vi "extract ROI.vi"(7 "ROI Descriptor":T2 {"Contours"."Type" items=["No Selection", "Point", "Line", "Rectangle", "Oval", "Polygon", "Freehand Region", "Annulus", "Unused2", "Unused3", "Broken Line", "Freehand Line", "Rotated Rectangle"]}, 10 "ROI ref in":T1, 11 "CCD image ref":T1) -> (0 "ROI SIZE":i32, 1 "Centroid XY":cluster{"X Centroid":sgl, "Y Centroid":sgl} {"Y Centroid" format="%.2f"; "X Centroid" format="%.2f"}, 3 "img_out":dbl[][](array[numeric]), 4 "Y_base":sgl, 6 "X_base":sgl)   [LabVIEW 2017]
doc: "本VI的作用是将已有的ROI提取出图像，计算出图心，然后在图心上标记ROI的序号。\n本VI对ROI的实际尺寸不敏感，可以随意修改。\n本VI由于最终要出图给camera window，因此不建议并行多分支执行，最好是先执行完，后续提取出来的图再分成各个分支并行执行。"
uses:
  <vilib>/vision/Image Controls.llb/IMAQ Image.ctl
  <vilib>/vision/NI_Vision_Development_Module.lvlib
  <vilib>/ptbypt/NI_PtbyPt.lvlib
  <vilib>/Analysis/NI_AALBase.lvlib
  <vilib>/Analysis/Matrix/NI_Matrix.lvlib
  <vilib>/Analysis/Matrix/Numeric/Multiply/Multiply - RM,R.vi
  <vilib>/Analysis/baseanly.llb/Normalize Matrix.vi
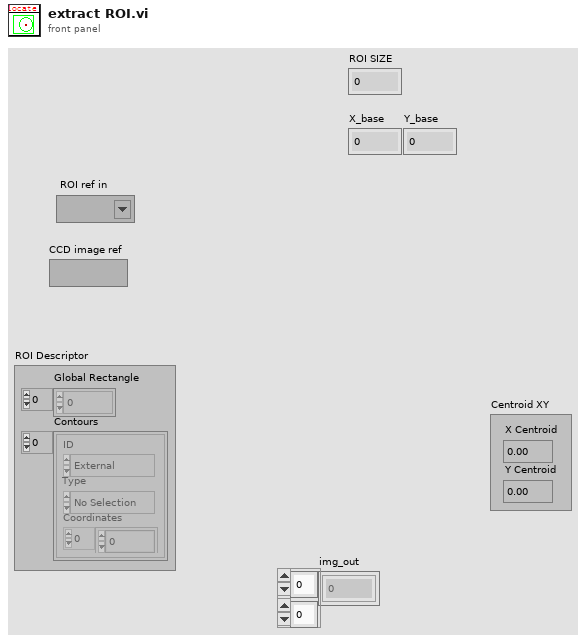
[diagram p1: front panel]
types:
  T1 = typedef "IMAQ Image.ctl" = refnum<image>
  T2 = typedef "ROI Descriptor" = cluster{"Global Rectangle":i32[], "Contours":cluster{"ID":enum32{"External", "Internal"}, "Type":u32, "Coordinates":i32[]}[]}
  T3 = typedef "IMAQ Rectangle" = cluster{"Left":i32, "Top":i32, "Right":i32, "Bottom":i32, "Rotation":dbl}
  T4 = typedef "NI_Matrix.lvlib/RealMatrix.ctl" = dbl[][]
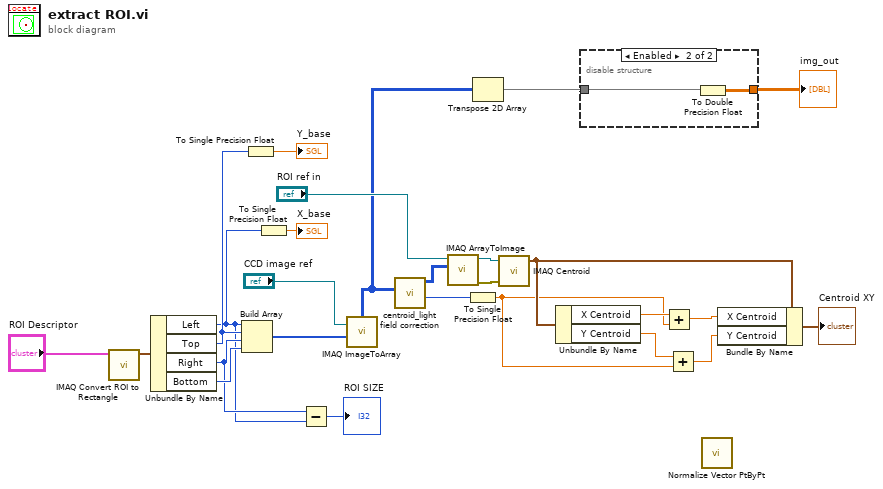
[diagram p0: block diagram]
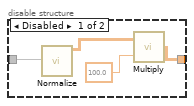
[diagram p2: hidden frame]
diagram:
  n1 = call "IMAQ Convert ROI to Rectangle"("ROI Descriptor"="ROI Descriptor") -> ("Rectangle"=w25:T3)  [unwired: 8 in, 1 out]
  n2 = Unbundle By Name(w25) -> ("Left"=w7:i32, "Top"=w22:i32, "Right"=w8:i32, "Bottom"=w24:i32)
  n3 = Build Array(w7, w22, w8, w24) -> (w23:i32[])
  n4 = To Single Precision Float(number=w22) -> (single precision float=→"Y_base":sgl)
  n5 = To Single Precision Float(number=w7) -> (single precision float=→"X_base":sgl)
  n6 = Subtract(x=w8, y=w7) -> (x-y=→"ROI SIZE":i32)
  n7 = call "IMAQ ImageToArray"("Optional Rectangle"=w23, "Image"="CCD image ref") -> ("Image Pixels (U8)"=w3:u8[][])  [unwired: 2 in, 4 out]
  n8 = call "centroid_light field correction.vi"("ROI array (no trans)"=w3) -> ("xybase core"=w13:i32, "ROI array out"=w17:u8[][])  [unwired: 9 in]
  n9 = call "IMAQ ArrayToImage"("Image Pixels (U8)"=w17, "Image"="ROI ref in") -> ("error out"=w18:errorcluster, "Image Out"=w5:T1)  [unwired: 8 in]
  n10 = To Single Precision Float(number=w13) -> (single precision float=w12:sgl)
  n11 = Transpose 2D Array(2D array=w3) -> (transposed array=w2:u8[][])
  n12 = call "IMAQ Centroid"("error in (no error)"=w18, "Image"=w5) -> ("Centroid"=w16:cluster{"X Centroid":sgl, "Y Centroid":sgl})  [unwired: 2 in, 1 out]
  n13 = Unbundle By Name(w16) -> ("X Centroid"=w15:sgl, "Y Centroid"=w14:sgl)
  n14 = disable-structure shown="Enabled" {
    disable-tunnel: w2 -> [w30 w32]
    disable-tunnel: [w27 w31] -> w1
    frame Disabled {
      n15 = call-poly <vilib>:"Normalize.vi"("Matrix"=w30) -> ("Normalized Matrix"=w28:T4)  [unwired: 1 in, 3 out]
      n16 = call-poly <vilib>:"Multiply.vi"("Real Scalar c"=100.0 ("y"), "Real Matrix A"=w28) -> ("A * c"=w27:T4)
    }
    frame Enabled {
      n17 = To Double Precision Float(number=w32) -> (double precision float=w31:dbl[][])
    }
  }
  "img_out" <- w1
  n18 = Add(x=w15, y=w12) -> (x+y=w11:sgl)
  n19 = Add(x=w14, y=w12) -> (x+y=w10:sgl)
  n20 = call <vilib>:"Normalize Vector PtByPt.vi"() -> ()  [unwired: 3 in, 4 out]
  n21 = Bundle By Name(cluster=w16, "X Centroid"=w11, "Y Centroid"=w10) -> (→"Centroid XY":cluster{"X Centroid":sgl, "Y Centroid":sgl})
